vi "Destination Tip Strip.vi"(8 "error in":errorcluster, 11 "SwitchMatrix in":refnum<class "SwitchMatrix.lvclass">) -> (0 "error out":errorcluster, 3 "SwitchMatrix out":refnum<class "SwitchMatrix.lvclass">)   [LabVIEW 2019, in "SwitchMatrix.lvlib" / "SwitchMatrix.lvclass"]
uses:
  Library/SwitchMatrix.lvclass
  Library/SwitchMatrix.lvclass/SwitchMatrix.ctl
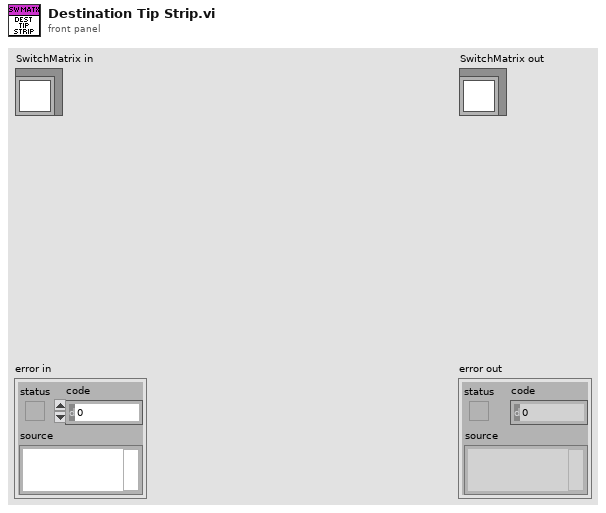
[diagram p1: front panel]
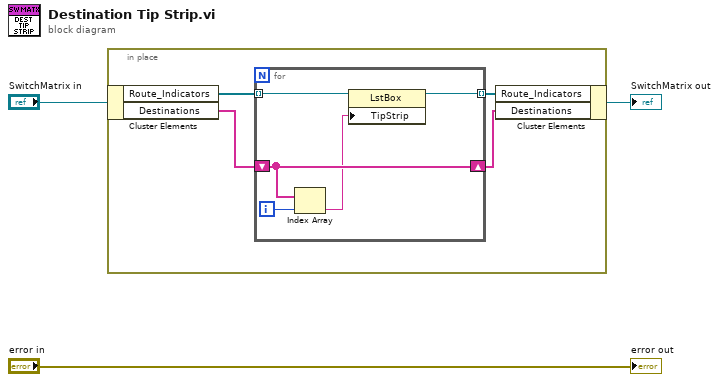
[diagram p0: block diagram]
diagram:
  n1 = in-place {
    n2 = in-place-cluster #1("SwitchMatrix in") -> ("Route_Indicators"=w7:refnum<vi>[], "Destinations"=w5:string[])
    n3 = for {
      tunnel: w7 -> [w12] mode=indexing
      tunnel: [w11] -> w6 mode=indexing
      shift-right: [w9] -> w4
      shift-left: w5 -> [w9]
      i -> [w10]
      n4 = Index Array(array=w9, index=w10) -> (element=w8:string)
      n5 = property class="LstBox"(reference=w12, "TipStrip"=w8) -> (reference out=w11:refnum<vi>)  [unwired: 1 in, 1 out]
    }
    n6 = in-place-cluster #1("Route_Indicators"=w6, "Destinations"=w4) -> (→"SwitchMatrix out":refnum<class "SwitchMatrix.lvclass">)
  }
  "error out" <- "error in"
